vi "Read Output.vi"(8 "error in (no error)":errorcluster, 10 "Channel (1: CH1)":i32(ring)=1 items=["CH1"=1, "CH2"=2], 11 "VISA resource name":refnum<visa-resource-name>) -> (0 "error out":errorcluster, 1 "Actual Current Level (A)":dbl, 2 "Actual Voltage Level (V)":dbl, 3 "VISA resource name out":refnum<visa-resource-name>)   [LabVIEW 2015, in "Siglent SPD3000 Series.lvlib"]
doc: "Returns the actual voltage level and actual current level for a desired channel."
uses:
  <instrlib>/Siglent SPD3000 Series/Siglent SPD3000 Series.lvlib
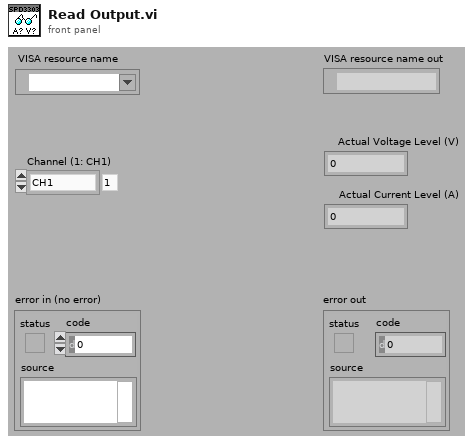
[diagram p1: front panel]
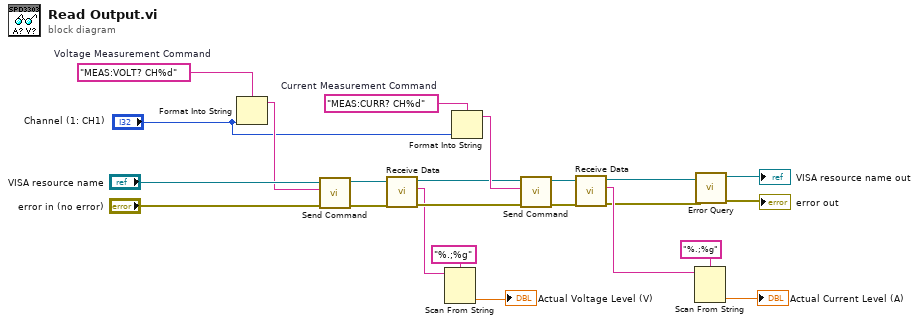
[diagram p0: block diagram]
diagram:
  w17 = "MEAS:CURR? CH%d"  # Current Measurement Command
  w19 = "MEAS:VOLT? CH%d"  # Voltage Measurement Command
  n1 = Format Into String(format string=w19, "Channel (1: CH1)") -> (resulting string=w18:string)  [unwired: 2 in, 1 out]
  n2 = call <instrlib>:"Send Command.vi"("error in (no error)"="error in (no error)", "Write Buffer (\"\")"=w18, "VISA resource name"="VISA resource name") -> ("error out"=w14:errorcluster, "VISA resource name out"=w15:refnum<visa-resource-name>)  [unwired: 7 in]
  n3 = call <instrlib>:"Receive Data.vi"("error in (no error)"=w14, "VISA resource name"=w15) -> ("error out"=w12:errorcluster, "Read Buffer"=w7:string, "VISA resource name out"=w13:refnum<visa-resource-name>)  [unwired: 6 in, 1 out]
  n4 = Scan From String(format string="%.;%g", input string=w7) -> (output 1=→"Actual Voltage Level (V)":dbl)  [unwired: 3 in, 3 out]
  n5 = Format Into String(format string=w17, "Channel (1: CH1)") -> (resulting string=w16:string)  [unwired: 2 in, 1 out]
  n6 = call <instrlib>:"Send Command.vi"("error in (no error)"=w12, "Write Buffer (\"\")"=w16, "VISA resource name"=w13) -> ("error out"=w10:errorcluster, "VISA resource name out"=w11:refnum<visa-resource-name>)  [unwired: 7 in]
  n7 = call <instrlib>:"Receive Data.vi"("error in (no error)"=w10, "VISA resource name"=w11) -> ("error out"=w2:errorcluster, "Read Buffer"=w6:string, "VISA resource name out"=w3:refnum<visa-resource-name>)  [unwired: 6 in, 1 out]
  n8 = Scan From String(format string="%.;%g", input string=w6) -> (output 1=→"Actual Current Level (A)":dbl)  [unwired: 3 in, 3 out]
  n9 = call <instrlib>:"Error Query.vi"("error in (no error)"=w2, "VISA resource name"=w3) -> ("error out"=→"error out":errorcluster, "VISA resource name out"=→"VISA resource name out":refnum<visa-resource-name>)  [unwired: 6 in, 2 out]
